vi "Drive Thru Obstacle (auto).vi"(7 "Drive through Obstacle":bool, 8 "Accelerometer":dbl, 9 "Speed":dbl, 10 "Gyro Value":dbl, 11 "Desired Angle":dbl format="%#_13g") -> (2 "Robot Drive Y":dbl, 3 "Robot Drive X":dbl)   [LabVIEW 2015]
uses:
  drive thru obstacle state.ctl
panel:
  out "Completed":bool
  in  "Robot Drive Forward":dbl=0.9 format="%#_13g"
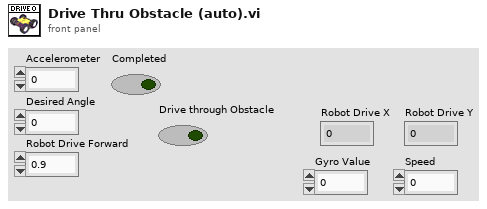
[diagram p1: front panel]
types:
  T1 = typedef "drive thru obstacle state.ctl" = enum16{"Ready", "Drive", "Correct position", "Complete"}
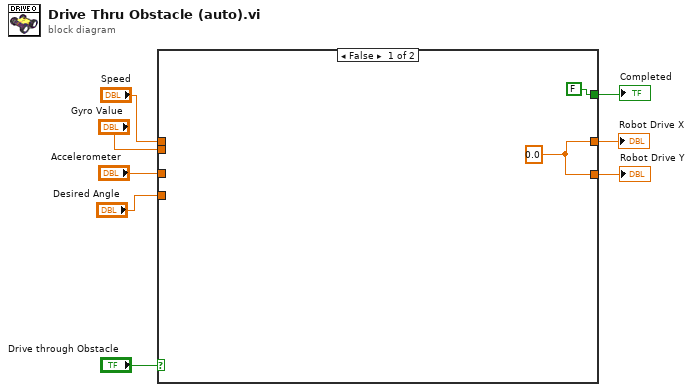
[diagram p0: block diagram]
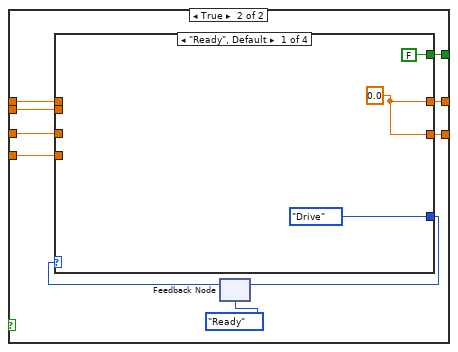
[diagram p2: hidden frame]
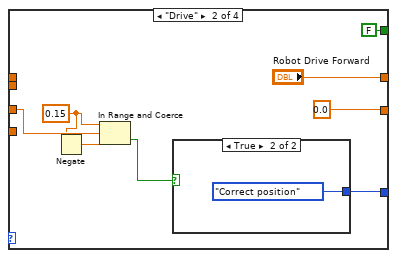
[diagram p3: hidden frame]
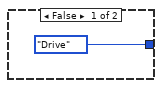
[diagram p4: hidden frame]
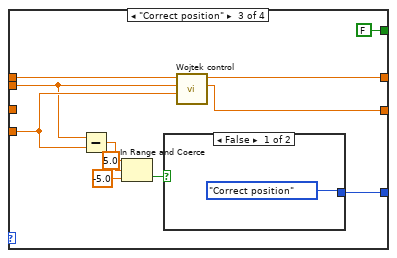
[diagram p5: hidden frame]
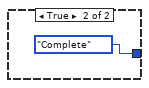
[diagram p6: hidden frame]
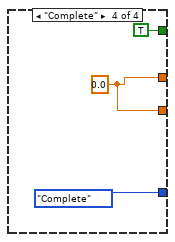
[diagram p7: hidden frame]
diagram:
  n1 = case shown="False" "Drive through Obstacle" {
    tunnel: [w10 w17] -> w7
    tunnel: [w10 w16] -> w6
    tunnel: "Gyro Value" -> [_ w15]
    tunnel: "Speed" -> [_ w14]
    tunnel: "Accelerometer" -> [_ w13]
    tunnel: "Desired Angle" -> [_ w12]
    tunnel: [FALSE w11] -> w1
    frame False {
      w10 = 0.0
    }
    frame True {
      n2 = feedback #1(drive_thru_obstacle_state."Ready") -> (w19:T1)
      n3 = case shown="\"Ready\", Default" w19 {
        tunnel: [drive_thru_obstacle_state."Drive" w31 w35 drive_thru_obstacle_state."Complete"] -> w18
        tunnel: [w22 "Robot Drive Forward" w43 w49] -> w17
        tunnel: [w22 0.0 w42 w49] -> w16
        tunnel: w15 -> [_ _ w40 _]
        tunnel: w14 -> [_ _ w44 _]
        tunnel: w13 -> [_ w28 _ _]
        tunnel: w12 -> [_ _ w41 _]
        tunnel: [FALSE FALSE FALSE TRUE] -> w11
        frame "Ready", Default {
          w22 = 0.0
        }
        frame "Drive" {
          w26 = 0.15 ("upper limit")
          n4 = Negate(x=w26) -> (-x=w27:dbl)
          n5 = In Range and Coerce(upper limit=w26, x=w28, lower limit=w27) -> (In Range?=w25:bool)  [unwired: 1 out]
          n6 = case shown="True" w25 {
            tunnel: [drive_thru_obstacle_state."Drive" drive_thru_obstacle_state."Correct position"] -> w31
            frame False {
            }
            frame True {
            }
          }
        }
        frame "Correct position" {
          n7 = Subtract(x=w40, y=w41) -> (x-y=w38:dbl)
          n8 = In Range and Coerce(upper limit=5.0, x=w38, lower limit=-5.0) -> (In Range?=w39:bool)  [unwired: 1 out]
          n9 = case shown="False" w39 {
            tunnel: [drive_thru_obstacle_state."Correct position" drive_thru_obstacle_state."Complete"] -> w35
            frame False {
            }
            frame True {
            }
          }
          n10 = call "Wojtek control.vi"("Desired Angle"=w41, "Gyro Angle"=w40, "Speed"=w44) -> ("right axis value"=w42:dbl, "left axis value"=w43:dbl)  [unwired: 7 in]
        }
        frame "Complete" {
          w49 = 0.0
        }
      }
      n11 = feedback-in #1(w18) -> ()
    }
  }
  "Robot Drive X" <- w7
  "Robot Drive Y" <- w6
  "Completed" <- w1
